vi "Result.vi"(8 "error in (no error)":errorcluster, 10 "Result":T1={"Name"="", "Message"="", "Description"="", "Status"=enum."Passed", "Result Type"=enum."Case", "Execution Time"=0.0}, 11 "Result Observer In":refnum<class "Result Observer.lvclass">) -> (0 "error out":errorcluster)   [LabVIEW 2020, in "Result Observer.lvclass"]
uses:
  Result Observer.lvclass
  Result/Result.ctl
  Result/Status.ctl
  Result/Type.ctl
  Result/Result.lvlib
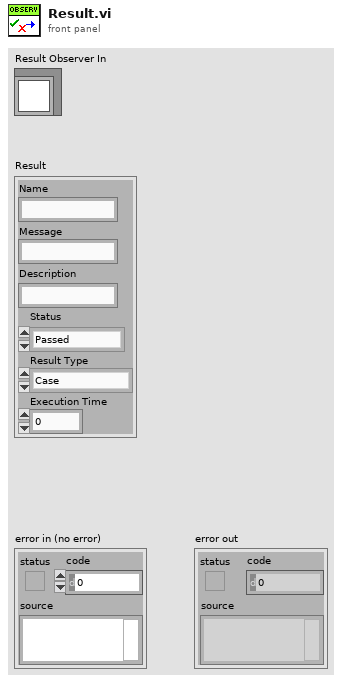
[diagram p1: front panel]
types:
  T1 = typedef "Result.lvlib/Result.ctl" = cluster{"Name":string, "Message":string, "Description":string, "Status":T2, "Result Type":T3, "Execution Time":dbl}
  T2 = typedef "Result.lvlib/Status.ctl" = enum16{"", "Passed", "Failed", "Error", "Skipped", "Setup Error", "Broken", "Teardown Error"}
  T3 = typedef "Result.lvlib/Type.ctl" = enum16{"Method", "Case", "Suite", "Pass", "Fail", "Skip", "Pass if", "Fail if", "Pass if Error", "Fail if Error", "Pass if Equal", "Fail if Equal"}
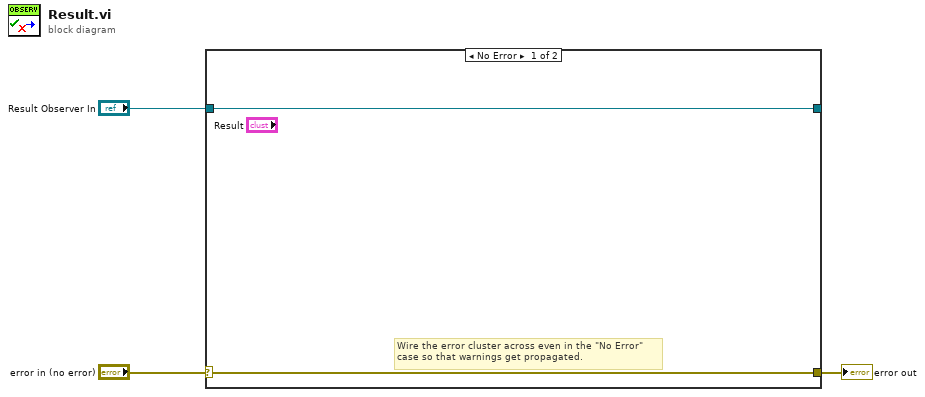
[diagram p0: block diagram]
diagram:
  n1 = case shown="No Error" "error in (no error)" {
    selector: "error in (no error)" -> [w4 w7]
    tunnel: [w4 w7] -> w2
    tunnel: [w5 w6] -> _
    tunnel: "Result Observer In" -> [w5 w6]
    frame No Error {
      # "Wire the error cluster across even in the \"No Error\"\ncase so that warnings get propagated."
    }
    frame Error {
    }
  }
  "error out" <- w2
